vi "Configure RemIO Module.vi"(8 "error in (no error)":errorcluster, 9 "Slave Ref In":refnum<k21>, 10 "11120 in":refnum<class "11120.lvclass">, 11 "Node Ptr In":T1 format="%.0x") -> (0 "error out":errorcluster, 1 "Slave Ref Out":refnum<k21>, 2 "11120 out":refnum<class "11120.lvclass">, 3 "Node Ptr Out":T1 format="%.0x")   [LabVIEW 2016, in "Modules.lvlib" / "11120.lvclass"]
uses:
  11120.lvclass
  <vilib>/NI Veristand/Custom Device API/Custom Device Item Ref.ctl
  11120.lvclass/11120.ctl
  <vilib>/Utility/error.llb/Error Cluster From Error Code.vi
  <vilib>/indcomecat/Remote IO/internal/_Configure REM-11120.vi
  <vilib>/ErrorRing/Error Ring.xnode
  <vilib>/indcomecat/Remote IO/NI ECAT Remote IO.lvlib
  <vilib>/NI Veristand/Custom Device API/Custom Device API.lvlib
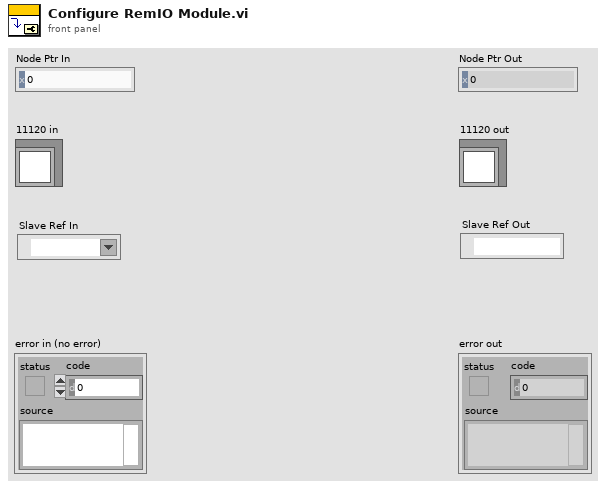
[diagram p1: front panel]
types:
  T1 = typedef "Custom Device API.lvlib/Custom Device Item Ref.ctl" = u64
  T2 = typedef "NI ECAT Remote IO.lvlib/mounting position REM-11120.ctl" = u8
  T3 = typedef "NI ECAT Remote IO.lvlib/channel number REM-11120.ctl" = u8
  T4 = typedef "NI ECAT Remote IO.lvlib/input filter time REM-11120.ctl" = u8
  T5 = typedef "NI ECAT Remote IO.lvlib/cold junction type REM-11120.ctl" = u8
  T6 = typedef "NI ECAT Remote IO.lvlib/resolution REM-11120.ctl" = u8
  T7 = typedef "NI ECAT Remote IO.lvlib/sensor type REM-11120.ctl" = u8
  T8 = cluster{"mounting position":T2, "parameters for channels":cluster{"channel number":T3, "input filter time":T4, "cold junction type":T5, "resolution":T6, "sensor type":T7}[]}
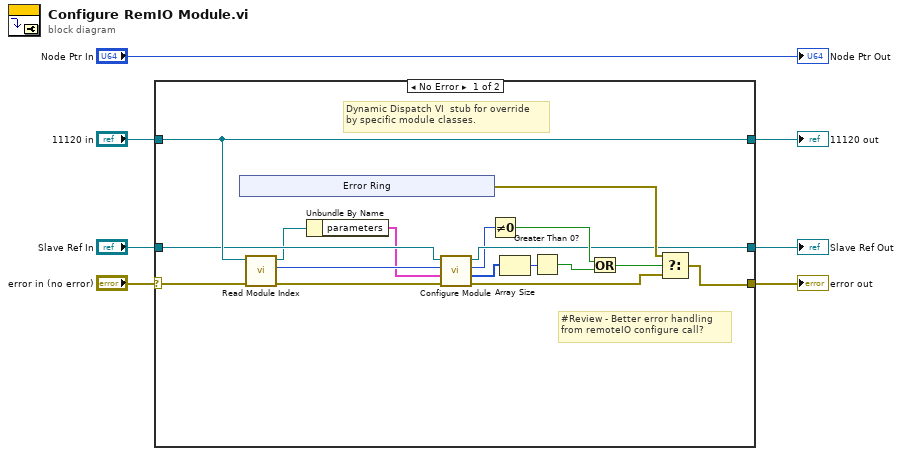
[diagram p0: block diagram]
diagram:
  n1 = case shown="No Error" "error in (no error)" {
    selector: "error in (no error)" -> [w20 w32]
    tunnel: [w21 w32] -> w1
    tunnel: [w18 w31] -> w3
    tunnel: "11120 in" -> [w18 w31]
    tunnel: [w14 w30] -> w2
    tunnel: "Slave Ref In" -> [w13 w30]
    frame No Error {
      # "#Review - Better error handling\nfrom remoteIO configure call?"
      # "Dynamic Dispatch VI  stub for override\nby specific module classes."
      n2 = xnode "Error Ring"() -> ("error out"=w22:errorcluster)
      n3 = call-dynamic "Read Module Index.vi"("error in (no error)"=w20, "RemIO Module in"=w18) -> ("error out"=w19:errorcluster, "Module Index"=w12:u8, "RemIO Module out"=w9:refnum<class "11120.lvclass">)  [unwired: 7 in]
      n4 = Unbundle By Name(w9) -> ("parameters"=w8:T8)
      n5 = call-poly <vilib>:"Configure Module.vi"("error in (no error)"=w19, "parameters"=w8, "module slot index"=w12, "slave reference in"=w13) -> ("error out"=w15:errorcluster, "negative confirmation"=w10:u8[], "SDO abort code"=w11:u32, "slave reference out"=w14:refnum<k21>)  [unwired: 4 in]
      n6 = Not Equal To 0?(x=w11) -> (x != 0?=w16:bool)
      n7 = Array Size(array=w10) -> (size(s)=w24:i32)
      n8 = Greater Than 0?(x=w24) -> (x > 0?=w23:bool)
      n9 = Or(x=w16, y=w23) -> (x .or. y?=w17:bool)
      n10 = Select(t=w22, s=w17, f=w15) -> (s? t:f=w21:errorcluster)
    }
    frame Error {
    }
  }
  "error out" <- w1
  "11120 out" <- w3
  "Slave Ref Out" <- w2
  "Node Ptr Out" <- "Node Ptr In"
